vi "save_subVI.vi"(2 "input cluster":errorcluster, 3 "array":string[](array[string]), 4 "Nome file":string="audio.log") -> (0 "File salvato in":path, 1 "t0":timestamp[](array[timestamp]))   [LabVIEW 2018]
uses:
  <vilib>/Utility/file.llb/Write Delimited Spreadsheet (string).vi
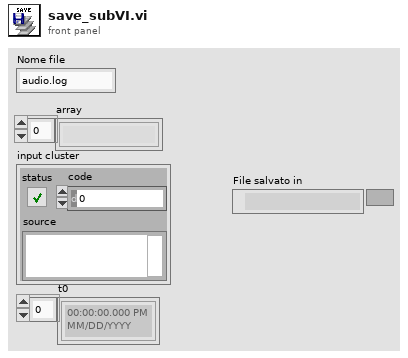
[diagram p1: front panel]
types:
  T1 = cluster{"t0[0]":timestamp, "t0[1]":timestamp, "t0[2]":timestamp, "t0[3]":timestamp, "t0[4]":timestamp, "t0[5]":timestamp, "t0[6]":timestamp, "t0[7]":timestamp, "t0[8]":timestamp}
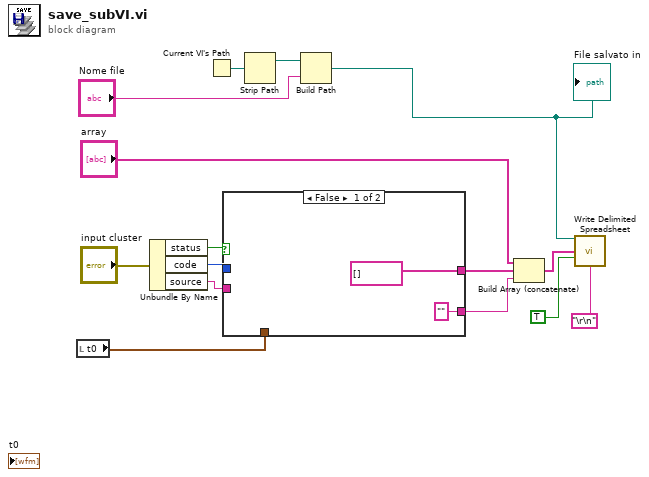
[diagram p0: block diagram]
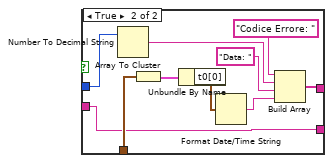
[diagram p2: hidden frame]
diagram:
  n1 = local read "t0"() -> (w3:timestamp[])
  n2 = Unbundle By Name("input cluster") -> ("status"=w8:bool, "code"=w7:i32, "source"=w2:string)
  n3 = Current VI's Path() -> (path=w12:path)
  n4 = case shown="False" w8 {
    tunnel: w7 -> [_ w27]
    tunnel: [string[] [] w24] -> w6
    tunnel: w3 -> [_ w19]
    tunnel: w2 -> [_ w18]
    tunnel: ["" ("source") w18] -> w1
    frame False {
    }
    frame True {
      n5 = Number To Decimal String(number=w27) -> (decimal integer string=w25:string)  [unwired: 1 in]
      n6 = Array To Cluster(array=w19) -> (cluster=w22:T1)
      n7 = Unbundle By Name(w22) -> ("t0[0]"=w21:timestamp)
      n8 = Format Date/Time String(seconds (now)=w21) -> (date/time string=w20:string)  [unwired: 2 in]
      n9 = Build Array("Codice Errore: " ("element"), w25, "Data: " ("element"), w20) -> (w24:string[])
    }
  }
  n10 = Strip Path(path=w12) -> (stripped path=w14:path)  [unwired: 1 out]
  n11 = Build Path(base path=w14, name or relative path="Nome file") -> (appended path=w13:path)
  "File salvato in" <- w13
  n12 = Build Array (concatenate)("array", w6, w1) -> (w9:string[])
  n13 = call-poly <vilib>:"Write Delimited Spreadsheet.vi"("file path (dialog if empty)"=w13, "1D data"=w9, "append to file? (new file:F)"=TRUE ("Concatena Log"), "delimiter (\\t)"="\r\n") -> ()  [unwired: 10 in, 2 out]
